vi "Get Overflow from FXP.vi"(5 "data in":fxp<+/-,18,1>[](array[numeric])=[0.0, 0.0, 0.0, 0.0, 0.0, 0.0, 0.0, 0.0, 0.0, 0.0, 0.0, 0.0, 0.0, 0.0, 0.0, 0.0]) -> (6 "overflow out":bool[](array[boolean]))   [LabVIEW 2018, in "GettingStarted_5774_FPGA.lvlib"]
doc: "Tracks the overflow status.\n\nA rising edge on the <B>latch overflow status</B> input updates the <B>overflow detected</B> output: this output is set to true if an overflow was detected since the last update."
uses:
  GettingStarted_5774_FPGA.lvlib
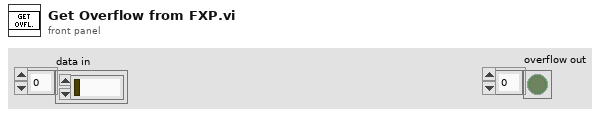
[diagram p1: front panel]
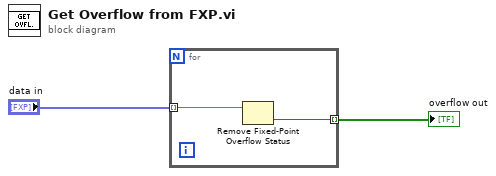
[diagram p0: block diagram]
diagram:
  n1 = for {
    tunnel: "data in" -> [w4] mode=indexing
    tunnel: [w3] -> w1 mode=indexing
    n2 = Remove Fixed-Point Overflow Status(3:w4) -> (0:w3:bool)  [unwired: 1 out]
  }
  "overflow out" <- w1
